vi "group Sync Read Add Param.vi"(10 "id":u8, 11 "group_num":i32) -> (3 "function return":u8)   [LabVIEW 2016, in "dxl_x86_c.lvlib"]
doc: "WINDECLSPEC uint8_t groupSyncReadAddParam (int group_num, uint8_t id);"
uses:
  dxl_x86_c.lvlib
  dxl_x86_c.dll
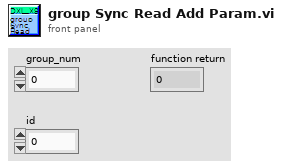
[diagram p1: front panel]
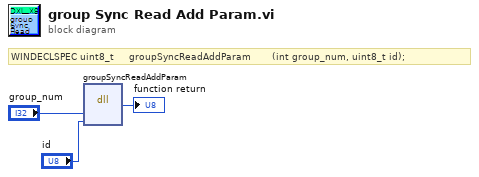
[diagram p0: block diagram]
diagram:
  # "WINDECLSPEC uint8_t     groupSyncReadAddParam       (int group_num, uint8_t id);"
  n1 = dll-call lib="C:/Users/Platform/Desktop/DynamixelSDK/labview/dxl_x86_c.lvlib/dxl_x86_c.*" fn="groupSyncReadAddParam"("group_num"="group_num", "id"="id") -> (→"function return":u8)  [unwired: 5 in, 2 out]
